vi "TDTRX6-Stop.vi"(11 "error in (no error)":errorcluster) -> (15 "error out":errorcluster)   [LabVIEW 2020]
doc: "Sets global variables that terminate the main DAQ loop."
uses:
  TDT-Signal Bank Action.ctl
  TDT-Globals.vi
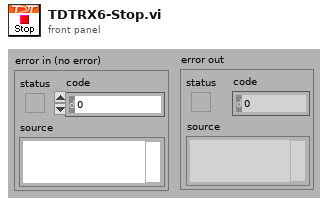
[diagram p1: front panel]
types:
  T1 = typedef "TDT-Signal Bank Action.ctl" = enum16{"Init", "Write", "Read", "Rewrite", "Reset", "Recycle", "Ramp up", "Ramp down", "Zero"}
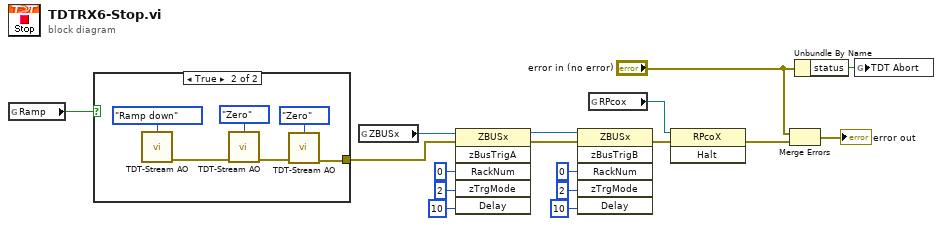
[diagram p0: block diagram]
diagram:
  n1 = global read "TDT-Globals.vi" "Ramp"() -> (w3:bool)
  n2 = case shown="True" w3 {
    tunnel: [_ w18] -> w4
    frame False {
    }
    frame True {
      n3 = call "TDT-Stream AO.vi"("Action"=TDT-Signal_Bank_Action."Ramp down") -> ("error out"=w20:errorcluster)  [unwired: 14 in]
      n4 = call "TDT-Stream AO.vi"("Action"=TDT-Signal_Bank_Action."Zero", "error in (no error)"=w20) -> ("error out"=w19:errorcluster)  [unwired: 13 in]
      n5 = call "TDT-Stream AO.vi"("Action"=TDT-Signal_Bank_Action."Zero", "error in (no error)"=w19) -> ("error out"=w18:errorcluster)  [unwired: 13 in]
    }
  }
  n6 = global read "TDT-Globals.vi" "ZBUSx"() -> (w14:refnum<k7>)
  n7 = invoke class="ZBUSx" method="zBusTrigA"(reference=w14, error in=w4, "RackNum"=0, "zTrgMode"=2, "Delay"=10) -> (reference out=w6:refnum<k7>, error out=w5:errorcluster)  [unwired: 1 in, 4 out]
  n8 = invoke class="ZBUSx" method="zBusTrigB"(reference=w6, error in=w5, "RackNum"=0, "zTrgMode"=2, "Delay"=10) -> (error out=w1:errorcluster)  [unwired: 1 in, 5 out]
  n9 = global read "TDT-Globals.vi" "RPcox"() -> (w2:refnum<k7>)
  n10 = invoke class="RPcoX" method="Halt"(reference=w2, error in=w1) -> (error out=w13:errorcluster)  [unwired: 1 in, 2 out]
  n11 = Merge Errors("error in (no error)", w13) -> (→"error out":errorcluster)
  n12 = Unbundle By Name("error in (no error)") -> ("status"=w10:bool)
  n13 = global write "TDT-Globals.vi" "TDT Abort"(w10) -> ()
